vi "set_config_cluster.vi"(8 "error in (no error)":errorcluster, 10 "config cluster variant":variant, 11 "DAQ_MG090622Camera in":refnum<class "DAQ_MG090622Camera.lvclass">) -> (0 "error out":errorcluster, 3 "DAQ_MG090622Camera out":refnum<class "DAQ_MG090622Camera.lvclass">)   [LabVIEW 2010, in "DAQ_MG090622Camera.lvclass"]
uses:
  DAQ_MG090622Camera.lvclass
  DAQ_MG090622Camera.lvclass/DAQ_MG090622Camera.ctl
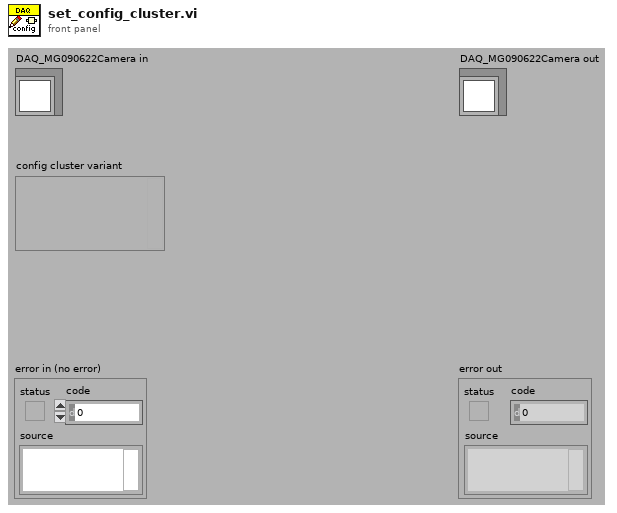
[diagram p1: front panel]
types:
  T1 = typedef "DAQ_MG090622Camera.lvclass/config_data_cluster.ctl" = cluster{"device name":string, "camera type":T2, "connection type":T3}
  T2 = typedef "DAQ_MG090622Camera.lvclass/camera_type_enum.ctl" = enum16{"gray scale", "RGB"}
  T3 = typedef "DAQ_MG090622Camera.lvclass/connection_type_enum.ctl" = enum16{"IEEE 1394 (FireWire)", "USB", "GigE", "CameraLink"}
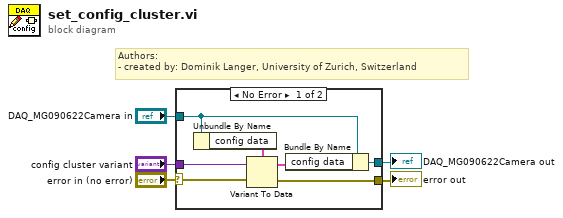
[diagram p0: block diagram]
diagram:
  # "Authors: \n- created by: Dominik Langer, University of Zurich, Switzerland"
  n1 = case shown="No Error" "error in (no error)" {
    selector: "error in (no error)" -> [w12 w13]
    tunnel: [w11 w13] -> w4
    tunnel: "DAQ_MG090622Camera in" -> [w7 w14]
    tunnel: "config cluster variant" -> [w9 _]
    tunnel: [w6 w14] -> w1
    frame No Error {
      n2 = Unbundle By Name(w7) -> ("config data"=w10:T1)
      n3 = Variant To Data(error in=w12, Variant=w9, type=w10) -> (error out=w11:errorcluster, data=w8:T1)
      n4 = Bundle By Name(cluster=w7, "config data"=w8) -> (w6:refnum<class "DAQ_MG090622Camera.lvclass">)
    }
    frame Error {
    }
  }
  "error out" <- w4
  "DAQ_MG090622Camera out" <- w1
